vi "Release.vi"(8 "Error In":errorcluster, 11 "Listeners In":refnum<queue>[](array[refnum])) -> (0 "Error Out":errorcluster, 3 "Listeners Out":refnum<queue>[](array[refnum]))   [LabVIEW 2025, in "LOGlib_LV2025.lvlib"]
uses:
  LOGlib_LV2025.lvlib
  Type Definitions/Statement.ctl
  Type Definitions/Tag.ctl
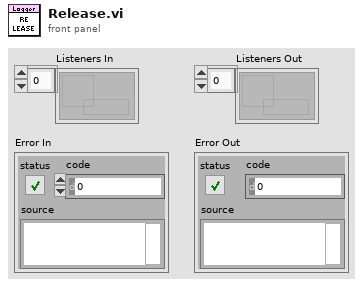
[diagram p1: front panel]
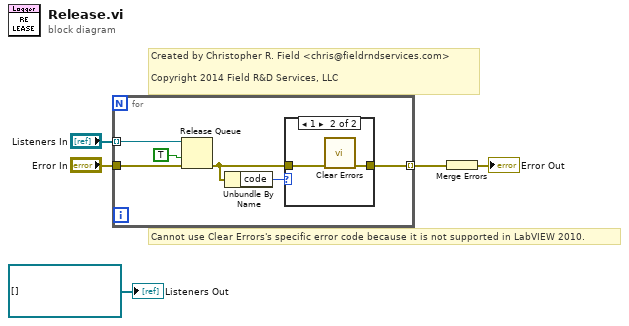
[diagram p0: block diagram]
diagram:
  # "Cannot use Clear Errors's specific error code because it is not supported in LabVIEW 2010."
  # "Created by Christopher R. Field <chris@fieldrndservices.com>\n\nCopyright 2014 Field R&D Services, LLC"
  n1 = for {
    tunnel: "Listeners In" -> [w11] mode=indexing
    tunnel: "Error In" -> [w10]
    tunnel: [w8] -> w1 mode=indexing
    n2 = Release Queue(queue=w11, force destroy? (F)=TRUE, error in (no error)=w10) -> (error out=w7:errorcluster)  [unwired: 2 out]
    n3 = Unbundle By Name(w7) -> ("code"=w6:i32)
    n4 = case shown="1" w6 {
      tunnel: [w12 w14] -> w8
      tunnel: w7 -> [w12 w13]
      frame 0, Default {
      }
      frame 1 {
        n5 = call <vilib>:"Clear Errors.vi"("error in (no error)"=w13) -> ("error out"=w14:errorcluster)  [unwired: 5 in, 1 out]
      }
    }
  }
  n6 = Merge Errors(w1) -> (→"Error Out":errorcluster)
  "Listeners Out" <- refnum<queue>[] [] ("Listeners Out")
